vi "诊断标定4.vi"(8 "CAN端口":u16(ring), 9 "设备索引号":u16(ring), 10 "CAN卡类型":u32(ring)=4) -> ()   [LabVIEW 2013] (continued)
            n2546 = property on="电流步长" class="DigNum (严格)"("Disabled"=w3724) -> ()  [unwired: 2 in, 2 out]
            n2547 = property on="SOC" class="DigNum (严格)"("Disabled"=0) -> ()  [unwired: 2 in, 2 out]
            n2548 = property on="充电总安时" class="DigNum (严格)"("Disabled"=w3723) -> ()  [unwired: 2 in, 2 out]
            n2549 = property on="放电总这时" class="DigNum (严格)"("Disabled"=w3723) -> ()  [unwired: 2 in, 2 out]
            n2550 = Not(x=w3731) -> (.not. x?=w3730:bool)
          }
          frame "车牌号" {
            w3734 = 2
            w3735 = 2
            w3737 = 2
            w3739 = 2
            w3742 = FALSE ("1 6")
            n2551 = property on="电池类型" class="DigNum (严格)"("Disabled"=w3739) -> ()  [unwired: 2 in, 2 out]
            n2552 = property on="电池厂家" class="DigNum (严格)"("Disabled"=w3739) -> ()  [unwired: 2 in, 2 out]
            n2553 = property on="电池地区" class="DigNum (严格)"("Disabled"=w3739) -> ()  [unwired: 2 in, 2 out]
            n2554 = property on="电池组序号" class="DigNum (严格)"("Disabled"=w3739) -> ()  [unwired: 2 in, 2 out]
            n2555 = property on="电池包串联数" class="DigNum (严格)"("Disabled"=w3739) -> ()  [unwired: 2 in, 2 out]
            n2556 = property on="电池包并联数" class="DigNum (严格)"("Disabled"=w3739) -> ()  [unwired: 2 in, 2 out]
            n2557 = property on="电池包安时数" class="DigNum (严格)"("Disabled"=w3739) -> ()  [unwired: 2 in, 2 out]
            n2558 = property on="电池组信息" class="Clust (严格)"("Disabled"=0) -> ()  [unwired: 2 in, 2 out]
            n2559 = property on="车牌号" class="Str"("Disabled"=0) -> ()  [unwired: 2 in, 2 out]
            n2560 = property on="电池包序号" class="DigNum (严格)"("Disabled"=2) -> ()  [unwired: 2 in, 2 out]
            n2561 = property on="充电次数" class="DigNum (严格)"("Disabled"=w3737) -> ()  [unwired: 2 in, 2 out]
            n2562 = property on="充满电时间" class="DigNum (严格)"("Disabled"=w3737) -> ()  [unwired: 2 in, 2 out]
            n2563 = property on="放空时间" class="DigNum (严格)"("Disabled"=w3737) -> ()  [unwired: 2 in, 2 out]
            n2564 = property on="最大允许单体电压" class="DigNum (严格)"("Disabled"=w3735) -> ()  [unwired: 2 in, 2 out]
            n2565 = property on="最大允许总电压" class="DigNum (严格)"("Disabled"=w3735) -> ()  [unwired: 2 in, 2 out]
            n2566 = property on="最大允许温度" class="DigNum (严格)"("Disabled"=w3735) -> ()  [unwired: 2 in, 2 out]
            n2567 = property on="最小允许温度" class="DigNum (严格)"("Disabled"=w3735) -> ()  [unwired: 2 in, 2 out]
            n2568 = property on="最大允许充电电流" class="DigNum (严格)"("Disabled"=w3735) -> ()  [unwired: 2 in, 2 out]
            n2569 = property on="最小允许充电电流" class="DigNum (严格)"("Disabled"=w3735) -> ()  [unwired: 2 in, 2 out]
            n2570 = property on="最小允许单体电压" class="DigNum (严格)"("Disabled"=w3735) -> ()  [unwired: 2 in, 2 out]
            n2571 = property on="电流步长" class="DigNum (严格)"("Disabled"=w3735) -> ()  [unwired: 2 in, 2 out]
            n2572 = property on="SOC" class="DigNum (严格)"("Disabled"=2) -> ()  [unwired: 2 in, 2 out]
            n2573 = property on="充电总安时" class="DigNum (严格)"("Disabled"=w3734) -> ()  [unwired: 2 in, 2 out]
            n2574 = property on="放电总这时" class="DigNum (严格)"("Disabled"=w3734) -> ()  [unwired: 2 in, 2 out]
            n2575 = Not(x=w3742) -> (.not. x?=w3741:bool)
          }
          frame "充电参数" {
            w3744 = 2
            w3745 = 0
            w3747 = 2
            w3749 = 2
            w3752 = FALSE ("1 6")
            n2576 = property on="电池类型" class="DigNum (严格)"("Disabled"=w3749) -> ()  [unwired: 2 in, 2 out]
            n2577 = property on="电池厂家" class="DigNum (严格)"("Disabled"=w3749) -> ()  [unwired: 2 in, 2 out]
            n2578 = property on="电池地区" class="DigNum (严格)"("Disabled"=w3749) -> ()  [unwired: 2 in, 2 out]
            n2579 = property on="电池组序号" class="DigNum (严格)"("Disabled"=w3749) -> ()  [unwired: 2 in, 2 out]
            n2580 = property on="电池包串联数" class="DigNum (严格)"("Disabled"=w3749) -> ()  [unwired: 2 in, 2 out]
            n2581 = property on="电池包并联数" class="DigNum (严格)"("Disabled"=w3749) -> ()  [unwired: 2 in, 2 out]
            n2582 = property on="电池包安时数" class="DigNum (严格)"("Disabled"=w3749) -> ()  [unwired: 2 in, 2 out]
            n2583 = property on="电池组信息" class="Clust (严格)"("Disabled"=0) -> ()  [unwired: 2 in, 2 out]
            n2584 = property on="车牌号" class="Str"("Disabled"=2) -> ()  [unwired: 2 in, 2 out]
            n2585 = property on="电池包序号" class="DigNum (严格)"("Disabled"=2) -> ()  [unwired: 2 in, 2 out]
            n2586 = property on="充电次数" class="DigNum (严格)"("Disabled"=w3747) -> ()  [unwired: 2 in, 2 out]
            n2587 = property on="充满电时间" class="DigNum (严格)"("Disabled"=w3747) -> ()  [unwired: 2 in, 2 out]
            n2588 = property on="放空时间" class="DigNum (严格)"("Disabled"=w3747) -> ()  [unwired: 2 in, 2 out]
            n2589 = property on="最大允许单体电压" class="DigNum (严格)"("Disabled"=w3745) -> ()  [unwired: 2 in, 2 out]
            n2590 = property on="最大允许总电压" class="DigNum (严格)"("Disabled"=w3745) -> ()  [unwired: 2 in, 2 out]
            n2591 = property on="最大允许温度" class="DigNum (严格)"("Disabled"=w3745) -> ()  [unwired: 2 in, 2 out]
            n2592 = property on="最小允许温度" class="DigNum (严格)"("Disabled"=w3745) -> ()  [unwired: 2 in, 2 out]
            n2593 = property on="最大允许充电电流" class="DigNum (严格)"("Disabled"=w3745) -> ()  [unwired: 2 in, 2 out]
            n2594 = property on="最小允许充电电流" class="DigNum (严格)"("Disabled"=w3745) -> ()  [unwired: 2 in, 2 out]
            n2595 = property on="最小允许单体电压" class="DigNum (严格)"("Disabled"=w3745) -> ()  [unwired: 2 in, 2 out]
            n2596 = property on="电流步长" class="DigNum (严格)"("Disabled"=w3745) -> ()  [unwired: 2 in, 2 out]
            n2597 = property on="SOC" class="DigNum (严格)"("Disabled"=w3744) -> ()  [unwired: 2 in, 2 out]
            n2598 = property on="充电总安时" class="DigNum (严格)"("Disabled"=w3744) -> ()  [unwired: 2 in, 2 out]
            n2599 = property on="放电总这时" class="DigNum (严格)"("Disabled"=w3744) -> ()  [unwired: 2 in, 2 out]
            n2600 = Not(x=w3752) -> (.not. x?=w3751:bool)
          }
          frame "假", Default {
            w3755 = FALSE ("1 6")
            n2601 = Not(x=w3755) -> (.not. x?=w3754:bool)
          }
        }
        n2602 = local write "等级 2"(w3505) -> ()
        n2603 = local write "1 6"(w3504) -> ()
        n2604 = local write "1 7"(w3503) -> ()
        n2605 = local write "1 8"(w3502) -> ()
        n2606 = local write "1 9"(w3501) -> ()
        n2607 = local write "1 10"(w3500) -> ()
        n2608 = property on="单个读取" class="Bool (严格)"("Visible"=w3499) -> ()  [unwired: 2 in, 2 out]
        n2609 = property on="单个写入" class="Bool (严格)"("Visible"=w3498) -> ()  [unwired: 2 in, 2 out]
      }
      event "从板个数": Value Change {
        n2610 = event-data() -> ()  [unwired: 7 out]
        n2611 = local read "从板个数"() -> (w3757:dbl)
        n2612 = call "多从板对应参数.vi"("从板个数"=w3757) -> ("输出数组"=w3758:string[])  [unwired: 1 in]
        n2613 = control-ref of="项目信息"() -> (w3759:refnum<vi>)
        n2614 = stacked-sequence {
          tunnel: w3759 -> [w3762 w3766 w3770]
          tunnel: w3758 -> [_ w3765 w3769]
          frame #0 {
            n2615 = invoke class="Tbl (严格)" method="Reinit To Default"(reference=w3762) -> ()  [unwired: 2 in, 3 out]
          }
          frame #1 {
            n2616 = call "表格数据输入-8.6.vi"("行数"=u32 0, "列数"=u32 0, "字符串数组"=w3765, "表格引用"=w3766) -> ()  [unwired: 8 out]
          }
          frame #2 {
            n2617 = Array Size(array=w3769) -> (size(s)=w3768:i32)
            n2618 = for {
              N: w3768 -> [_]
              tunnel: [""] -> w3767 mode=indexing
            }
            n2619 = call "表格数据输入-8.6.vi"("行数"=u32 0, "列数"=u32 1, "字符串数组"=w3767, "表格引用"=w3770) -> ()  [unwired: 8 out]
          }
        }
      }
      event "主界面选项": Value Change {
        n2620 = event-data() -> ("NewVal"=w3774:enum32{"单选选项1", "单选选项2", "单选选项2 2", "单选选项2 3"})  [unwired: 6 out]
        n2621 = control-ref of="单选选项2 2"() -> (w3779:refnum<vi>)
        n2622 = control-ref of="单选选项2"() -> (w3781:refnum<vi>)
        n2623 = control-ref of="单选选项1"() -> (w3780:refnum<vi>)
        n2624 = control-ref of="单选选项2 3"() -> (w3775:refnum<vi>)
        n2625 = Build Array(w3780, w3781, w3779, w3775) -> (w3778:refnum<vi>[])
        n2626 = case shown="\"单选选项2 3\"" w3774 {
          selector: w3774 -> [w3792 w3797 w3802 w3807]
          tunnel: w3778 -> [w3793 w3798 w3803 w3808]
          tunnel: [w3791 w3796 w3801 w3806] -> w3784
          tunnel: [w3790 w3795 w3800 w3805] -> w3783
          tunnel: [enum32{"读写参数", "版本读取", "其它诊断"}."读写参数" ("选项卡控件 2") enum32{"读写参数", "版本读取", "其它诊断"}."版本读取" ("选项卡控件 2") enum32{"读写参数", "版本读取", "其它诊断"}."其它诊断" ("选项卡控件 2") enum32{"读写参数", "版本读取", "其它诊断", "高压板校正"}."高压板校正" ("选项卡控件 2")] -> w3782
          frame "单选选项1", Default {
            n2627 = Delete From Array(array=w3793, index=w3792) -> (deleted portion=w3790:refnum<vi>, array with subset deleted=w3791:refnum<vi>[])  [unwired: 1 in]
          }
          frame "单选选项2" {
            n2628 = Delete From Array(array=w3798, index=w3797) -> (deleted portion=w3795:refnum<vi>, array with subset deleted=w3796:refnum<vi>[])  [unwired: 1 in]
          }
          frame "单选选项2 2" {
            n2629 = Delete From Array(array=w3803, index=w3802) -> (deleted portion=w3800:refnum<vi>, array with subset deleted=w3801:refnum<vi>[])  [unwired: 1 in]
          }
          frame "单选选项2 3" {
            n2630 = Delete From Array(array=w3808, index=w3807) -> (deleted portion=w3805:refnum<vi>, array with subset deleted=w3806:refnum<vi>[])  [unwired: 1 in]
          }
        }
        n2631 = local write "选项卡控件 2"(w3782) -> ()
        n2632 = for {
          tunnel: u32 16777215 -> [w3788]
          tunnel: w3784 -> [w3787] mode=indexing
          n2633 = property class="Bool (严格)"(reference=w3787, "BoolText.TextColor"=w3788) -> ()  [unwired: 1 in, 2 out]
        }
        n2634 = property class="Bool (严格)"(reference=w3783, "BoolText.TextColor"=u32 87470) -> ()  [unwired: 1 in, 2 out]
      }
      event "主从板": Value Change {
        n2635 = event-data() -> ()  [unwired: 7 out]
        n2636 = control-ref of="单选选项2"() -> (w3816:refnum<vi>)
        n2637 = control-ref of="单选选项1"() -> (w3815:refnum<vi>)
        n2638 = local read "主从板"() -> (w3823:enum32{"单选选项2", "单选选项1"})
        n2639 = Build Array(w3816, w3815) -> (w3822:refnum<vi>[])
        n2640 = case shown="\"单选选项2\"" w3823 {
          selector: w3823 -> [w3867 w3892]
          tunnel: w3822 -> [w3868 w3891]
          tunnel: [enum32{"主板", "从板"}."主板" ("主从选择") enum32{"主板", "从板"}."从板" ("主从选择")] -> w3821
          tunnel: [w3866 w3890] -> w3818
          tunnel: [w3865 w3889] -> w3817
          tunnel: [TRUE FALSE] -> w3813
          tunnel: [w3826 w3869] -> w3810
          tunnel: [w3827 w3874] -> w3809
          frame "单选选项1", Default {
            n2641 = global read "功能码全局.vi" "主板项目信息7"() -> (w3838:bool[])
            n2642 = global read "功能码全局.vi" "主板控制类信息10"() -> (w3842:bool[])
            n2643 = global read "功能码全局.vi" "主板故障阀值9"() -> (w3839:bool[])
            n2644 = global read "功能码全局.vi" "主板项目信息5"() -> (w3852:bool[])
            n2645 = global read "功能码全局.vi" "主板项目信息6"() -> (w3862:bool[])
            n2646 = global read "功能码全局.vi" "主板项目信息4"() -> (w3861:bool[])
            n2647 = global read "功能码全局.vi" "主板版本号11"() -> (w3853:bool[])
            n2648 = Delete From Array(array=w3862, length=1 ("长度"), index=0 ("索引")) -> (deleted portion=w3851:bool[], array with subset deleted=w3834:bool[])
            n2649 = Index Array(array=w3861, index #1=5 ("索引"), index #2=6 ("索引")) -> (element #1=w3850:bool, element #2=w3833:bool)
            n2650 = Index Array(array=w3853) -> (element #1=w3846:bool, element #2=w3829:bool)  [unwired: 2 in]
            n2651 = Array Subset(array=w3839, index=2 ("索引"), length=3 ("长度")) -> (w3848:bool[])
            n2652 = Delete From Array(array=w3838, length=3 ("索引"), index=2 ("长度")) -> (deleted portion=w3849:bool[], array with subset deleted=w3832:bool[])
            n2653 = Array Subset(array=w3842, index=4 ("索引"), length=2 ("长度")) -> (w3847:bool[])
            n2654 = Delete From Array(array=w3868, index=w3867) -> (deleted portion=w3865:refnum<vi>, array with subset deleted=w3866:refnum<vi>[])  [unwired: 1 in]
            n2655 = Insert Into Array(array=w3852, new element #1=w3851, new element #2=w3850, new element #3=w3849, new element #4=w3848, new element #5=w3847, new element #6=w3846) -> (w3845:bool[])  [unwired: 1 in]
            n2656 = Array Subset(array=w3842, index=6 ("索引"), length=2 ("长度")) -> (w3830:bool[])
            n2657 = Array Subset(array=w3839, index=5 ("索引"), length=3 ("长度")) -> (w3831:bool[])
            n2658 = And Array Elements(Boolean array=w3845) -> (logical AND=w3827:bool)
            n2659 = Insert Into Array(array=w3834, new element #1=w3833, new element #2=w3832, new element #3=w3831, new element #4=w3830, new element #5=w3829) -> (w3828:bool[])  [unwired: 1 in]
            n2660 = And Array Elements(Boolean array=w3828) -> (logical AND=w3826:bool)
          }
          frame "单选选项2" {
            n2661 = global read "功能码全局.vi" "15"() -> (w3886:bool[])
            n2662 = global read "功能码全局.vi" "16"() -> (w3883:bool[])
            n2663 = Delete From Array(array=w3891, index=w3892) -> (deleted portion=w3889:refnum<vi>, array with subset deleted=w3890:refnum<vi>[])  [unwired: 1 in]
            n2664 = Index Array(array=w3883, index #1=4 ("索引"), index #2=5 ("索引"), index #3=6 ("索引"), index #4=7 ("索引")) -> (element #1=w3877:bool, element #2=w3876:bool, element #3=w3872:bool, element #4=w3871:bool)
            n2665 = Delete From Array(array=w3886, length=4 ("长度"), index=0 ("索引")) -> (deleted portion=w3878:bool[], array with subset deleted=w3873:bool[])
            n2666 = Insert Into Array(array=w3873, new element #1=w3872, new element #2=w3871) -> (w3870:bool[])  [unwired: 1 in]
            n2667 = Insert Into Array(array=w3878, new element #1=w3877, new element #2=w3876) -> (w3875:bool[])  [unwired: 1 in]
            n2668 = And Array Elements(Boolean array=w3870) -> (logical AND=w3869:bool)
            n2669 = And Array Elements(Boolean array=w3875) -> (logical AND=w3874:bool)
          }
        }
        n2670 = property on="全部写入" class="Bool (严格)"("Visible"=w3810) -> ()  [unwired: 2 in, 2 out]
        n2671 = property on="全部读取" class="Bool (严格)"("Visible"=w3809) -> ()  [unwired: 2 in, 2 out]
        n2672 = property on="从板个数" class="DigNum (严格)"("Visible"=w3813) -> ()  [unwired: 2 in, 2 out]
        n2673 = local write "主从选择"(w3821) -> ()
        n2674 = for {
          tunnel: u32 87470 -> [w3825]
          tunnel: w3818 -> [w3824] mode=indexing
          n2675 = property class="Bool (严格)"(reference=w3824, "BoolText.TextColor"=w3825) -> ()  [unwired: 1 in, 2 out]
        }
        n2676 = Not(x=w3813) -> (.not. x?=w3814:bool)
        n2677 = property class="Bool (严格)"(reference=w3817, "BoolText.TextColor"=u32 16777215) -> ()  [unwired: 1 in, 2 out]
        n2678 = property on="主板选项" class="Tree (严格)"("Visible"=w3813) -> ()  [unwired: 2 in, 2 out]
        n2679 = property on="从板选项" class="Tree (严格)"("Visible"=w3814) -> ()  [unwired: 2 in, 2 out]
        n2680 = property on="当前从板板号" class="DigNum (严格)"("Visible"=w3814) -> ()  [unwired: 2 in, 2 out]
      }
      event "从板板号": Value Change {
        n2681 = event-data() -> ()  [unwired: 7 out]
        n2682 = local read "key names"() -> (w3894:string[])
        n2683 = Empty Array?(array=w3894) -> (empty?=w3893:bool)
        n2684 = case shown="假" w3893 {
          tunnel: w3894 -> [w3897 _]
          frame False {
            n2685 = stacked-sequence {
              seq-local: [w3898 _] -> [_ w3961]
              tunnel: w3897 -> [w3906 _]
              frame #0 {
                w3937 = 2 ("长度")
                w3934 = 20 ("长度")
                w3922 = 1 ("索引")
                n2686 = local read "从板板号"() -> (w3898:u8)
                n2687 = local read "输出数组"() -> (w3907:string[][])
                n2688 = Decrement(x=w3898) -> (x-1=w3904:u8)
                n2689 = Index Array(array=w3907, index (col)=w3904) -> (element=w3935:string[])  [unwired: 1 in]
                n2690 = global write "读配置文件全局2.vi" "从板板号"(w3898) -> ()
                n2691 = Search 1D Array(1D array=w3906, element="风机开启温度" ("元素")) -> (index of element=w3919:i32)  [unwired: 1 in]
                n2692 = Search 1D Array(1D array=w3906, element="电压过高一级" ("元素"), start index (0)=w3919) -> (index of element=w3917:i32)
                n2693 = Decrement(x=w3919) -> (x-1=w3921:i32)
                n2694 = Array Subset(array=w3935, index=w3922, length=w3921) -> (w3905:string[])
                n2695 = Array Subset(array=w3935, index=w3917, length=21 ("长度")) -> (w3909:string[])
                n2696 = Array Subset(array=w3906, index=w3922, length=w3921) -> (w3952:string[])
                n2697 = Array Subset(array=w3935, index=w3919, length=7 ("长度")) -> (w3915:string[])
                n2698 = for {
                  tunnel: w3909 -> [w3954] mode=indexing
                  tunnel: [w3953] -> w3908 mode=indexing
                  n2699 = Fract/Exp String To Number(string=w3954) -> (number=w3953:dbl)  [unwired: 3 in, 1 out]
                }
                n2700 = for {
                  tunnel: w3915 -> [w3956] mode=indexing
                  tunnel: [w3955] -> w3899 mode=indexing
                  n2701 = Fract/Exp String To Number(string=w3956) -> (number=w3955:dbl)  [unwired: 3 in, 1 out]
                }
                n2702 = Delete From Array(array=w3908, length=7 ("长度"), index=0 ("索引")) -> (deleted portion=w3902:dbl[], array with subset deleted=w3912:dbl[])
                n2703 = Array To Cluster(array=w3899) -> (cluster=w3924:T23)
                n2704 = global write "读配置文件全局2.vi" "加热控制参数"(w3899) -> ()
                n2705 = Delete From Array(array=w3912, length=7 ("长度"), index=0 ("索引")) -> (deleted portion=w3901:dbl[], array with subset deleted=w3900:dbl[])
                n2706 = local write "加热控制参数"(w3924) -> ()
                n2707 = Array To Cluster(array=w3902) -> (cluster=w3949:T23)
                n2708 = Array To Cluster(array=w3900) -> (cluster=w3951:T23)
                n2709 = Array To Cluster(array=w3901) -> (cluster=w3950:T23)
                n2710 = global write "读配置文件全局2.vi" "三级故障阀值"(w3900) -> ()
                n2711 = global write "读配置文件全局2.vi" "一级故障阀值"(w3902) -> ()
                n2712 = global write "读配置文件全局2.vi" "二级故障阀值"(w3901) -> ()
                n2713 = local write "一级故障 6"(w3949) -> ()
                n2714 = local write "一级故障 8"(w3951) -> ()
                n2715 = local write "一级故障 7"(w3950) -> ()
                n2716 = Search 1D Array(1D array=w3952, element="温度个数" ("元素")) -> (index of element=w3931:i32)  [unwired: 1 in]
                n2717 = Search 1D Array(1D array=w3952, element="第一个保险通道" ("元素")) -> (index of element=w3932:i32)  [unwired: 1 in]
                n2718 = Search 1D Array(1D array=w3952, element="电压个数" ("元素")) -> (index of element=w3930:i32)  [unwired: 1 in]
                n2719 = Search 1D Array(1D array=w3952, element="第1通道电压个数" ("元素")) -> (index of element=w3933:i32)  [unwired: 1 in]
                n2720 = Array Subset(array=w3905, index=w3930, length=2 ("长度")) -> (w3938:string[])
                n2721 = Array Subset(array=w3905, index=w3931, length=w3937) -> (w3940:string[])
                n2722 = Array Subset(array=w3905, index=w3932, length=20 ("长度")) -> (w3941:string[])
                n2723 = Array Subset(array=w3905, index=w3933, length=w3934) -> (w3939:string[])
                n2724 = Insert Into Array(array=w3938, new element #1=w3939, new element #2=w3940, new element #3=w3941) -> (w3903:string[])  [unwired: 1 in]
                n2725 = Array Subset(array=w3952, index=w3930, length=w3937) -> (w3942:string[])
                n2726 = Array Subset(array=w3952, index=w3931, length=w3937) -> (w3944:string[])
                n2727 = Array Subset(array=w3952, index=w3932, length=w3934) -> (w3945:string[])
                n2728 = Array Subset(array=w3952, index=w3933, length=w3934) -> (w3943:string[])
                n2729 = global write "读配置文件全局2.vi" "表格"(w3903) -> ()
                n2730 = Insert Into Array(array=w3942, new element #1=w3943, new element #2=w3944, new element #3=w3945) -> (w3947:string[])  [unwired: 1 in]
                n2731 = Build Array(w3947, w3903) -> (w3946:string[][])
                n2732 = Transpose 2D Array(2D array=w3946) -> (transposed array=w3948:string[][])
                n2733 = local write "项目信息 2"(w3948) -> ()
              }
              frame #1 {
                n2734 = Number To Decimal String(number=w3961) -> (decimal integer string=w3959:string)  [unwired: 1 in]
                n2735 = control-ref of="结果"() -> (w3964:refnum<vi>)
                n2736 = Concatenate Strings("从板", w3959, "导入完成") -> (w3957:string)
                n2737 = Build Array(w3957) -> (w3962:string[])
                n2738 = call "表格编辑.vi"("新元素/子数组"=w3962, "活动单元格:单元格背景色"=u32 6618880, "MCListbox引用句柄"=w3964) -> ()  [unwired: 9 out]
              }
            }
          }
          frame True {
          }
        }
      }
      event "读配置文件": Value Change {
        n2739 = event-data() -> ("NewVal"=w3965:bool)  [unwired: 6 out]
        n2740 = case shown="真" w3965 {
          tunnel: w3969 -> [w3971 w3977]
          tunnel: [w3971 w3976] -> w3968
          tunnel: w3967 -> [w3970 w3975]
          tunnel: [w3970 w3974] -> w3966
          frame False {
          }
          frame True {
            n2741 = local write "布尔"(TRUE ("布尔")) -> ()
            n2742 = Enqueue Element(queue=w3977, element="读配置文件", error in (no error)=w3975) -> (queue out=w3976:refnum<queue>, error out=w3974:errorcluster)  [unwired: 2 out]
            n2743 = call <vilib>:"Set Busy.vi"() -> ()  [unwired: 4 in, 8 out]
          }
        }
      }
      event "写配置文件": Value Change {
        n2744 = event-data() -> ("NewVal"=w3978:bool)  [unwired: 6 out]
        n2745 = case shown="真" w3978 {
          tunnel: w3982 -> [w3984 w3989]
          tunnel: [w3984 w3988] -> w3981
          tunnel: w3980 -> [w3983 w3987]
          tunnel: [w3983 w3986] -> w3979
          frame False {
          }
          frame True {
            n2746 = call <vilib>:"Set Busy.vi"() -> ()  [unwired: 4 in, 8 out]
            n2747 = Enqueue Element(queue=w3989, element="写配置文件", error in (no error)=w3987) -> (queue out=w3988:refnum<queue>, error out=w3986:errorcluster)  [unwired: 2 out]
          }
        }
      }
      event "继电器全开": Value Change {
        n2748 = event-data() -> ("NewVal"=w3990:bool)  [unwired: 6 out]
        n2749 = stacked-sequence {
          tunnel: w3990 -> [_ w4000 _]
          frame #0 {
            w3993 = FALSE ("清BUFF")
            n2750 = local write "继电器超时处理"(FALSE ("继电器超时处理")) -> ()
            n2751 = local write "主从选择"(enum32{"主板", "从板"}."主板" ("主从选择")) -> ()
            n2752 = local write "正级继电器 12"(w3993) -> ()
            n2753 = local write "清BUFF"(w3993) -> ()
            n2754 = local write "正级继电器 2"(w3993) -> ()
            n2755 = local write "正级继电器 3"(w3993) -> ()
            n2756 = local write "正级继电器 4"(w3993) -> ()
            n2757 = local write "正级继电器 5"(w3993) -> ()
            n2758 = local write "正级继电器 6"(w3993) -> ()
          }
          frame #1 {
            n2759 = case shown="真" w4000 {
              selector: w4000 -> [_ w4015]
              frame False {
              }
              frame True {
                w4011 = 256.0 ("y")
                w4002 = u32 1 ("命令序号")
                w4001 = u8 192 ("命令")
                n2760 = local read "动作保持时间"() -> (w4012:dbl)
                n2761 = Quotient & Remainder(x=w4012, y=w4011) -> (x-y*floor(x/y)=w4004:dbl, floor(x/y)=w4008:dbl)
                n2762 = Quotient & Remainder(x=w4008, y=w4011) -> (x-y*floor(x/y)=w4005:dbl, floor(x/y)=w4009:dbl)
                n2763 = local read "设备索引号"() -> (w4019:u16)
                n2764 = Quotient & Remainder(x=w4009, y=w4011) -> (x-y*floor(x/y)=w4006:dbl, floor(x/y)=w4010:dbl)
                n2765 = local read "CAN卡类型"() -> (w4020:u32)
                n2766 = local read "CAN端口"() -> (w4018:u16)
                n2767 = Boolean To (0,1)(Boolean=w4015) -> (0, 1=w4013:i16)
                n2768 = Quotient & Remainder(x=w4010, y=w4011) -> (x-y*floor(x/y)=w4007:dbl)  [unwired: 1 out]
                n2769 = Build Array(i16 170 ("元素"), w4013, w4007, w4006, w4005, w4004, 0.0 ("元素")) -> (w4016:dbl[])
                n2770 = call "多帧发送机制(EV05).vi"("can卡类型"=w4020, "设备索引号"=w4019, "CAN端口"=w4018, "命令"=w4001, "板号"=u8 0, "命令序号"=w4002, "输入数据"=w4016) -> ()  [unwired: 1 in, 12 out]
                n2771 = local write "命令序号"(w4002) -> ()
                n2772 = local write "命令"(w4001) -> ()
              }
            }
            n2773 = local write "控制1"(TRUE ("控制1")) -> ()
            n2774 = local write "写?"(FALSE ("写?")) -> ()
            n2775 = global write "EV05全局变量1.vi" "流控帧 2"(FALSE ("流控帧 2")) -> ()
            n2776 = local write "消除"(TRUE ("消除")) -> ()
          }
          frame #2 {
            n2777 = flat-sequence {
              tunnel: [w4022] -> w4021
              tunnel: w4021 -> [w4029]
              frame #0 {
                n2778 = while {
                  tunnel: [w4023] -> w4022
                  i -> [w4027]
                  stop <- w4024 stop-if-true
                  n2779 = local read "继电器超时处理"() -> (w4023:bool)
                  n2780 = Greater Or Equal?(x=w4027, y=20) -> (x >= y?=w4025:bool)
                  n2781 = Wait Until Next ms Multiple(millisecond multiple=u32 100 ("毫秒倍数")) -> ()  [unwired: 1 out]
                  n2782 = Or(x=w4023, y=w4025) -> (x .or. y?=w4024:bool)
                }
              }
              frame #1 {
                n2783 = case shown="假" w4029 {
                  frame False {
                    n2784 = One Button Dialog(message="继电器处理超时" ("消息"), button name ("OK")="是" ("按钮名称（“确定”）")) -> ()  [unwired: 1 out]
                  }
                  frame True {
                    w4032 = TRUE ("清BUFF")
                    n2785 = local write "正级继电器 12"(w4032) -> ()
                    n2786 = local write "正级继电器 2"(w4032) -> ()
                    n2787 = local write "正级继电器 3"(w4032) -> ()
                    n2788 = local write "正级继电器 4"(w4032) -> ()
                    n2789 = local write "正级继电器 5"(w4032) -> ()
                    n2790 = local write "正级继电器 6"(w4032) -> ()
                  }
                }
              }
            }
          }
        }
      }
      event "继电器全关": Value Change {
        n2791 = event-data() -> ("NewVal"=w4033:bool)  [unwired: 6 out]
        n2792 = stacked-sequence {
          tunnel: w4033 -> [_ w4044 _]
          frame #0 {
            w4036 = TRUE ("清BUFF")
            n2793 = local write "正级继电器 12"(w4036) -> ()
            n2794 = local write "正级继电器 2"(w4036) -> ()
            n2795 = local write "正级继电器 3"(w4036) -> ()
            n2796 = local write "正级继电器 4"(w4036) -> ()
            n2797 = local write "正级继电器 5"(w4036) -> ()
            n2798 = local write "正级继电器 6"(w4036) -> ()
            n2799 = local write "继电器超时处理"(FALSE ("继电器超时处理")) -> ()
            n2800 = local write "主从选择"(enum32{"主板", "从板"}."主板" ("主从选择")) -> ()
            n2801 = local write "清BUFF"(FALSE ("清BUFF")) -> ()
          }
          frame #1 {
            n2802 = case shown="真" w4044 {
              selector: w4044 -> [_ w4059]
              frame False {
              }
              frame True {
                w4055 = 256.0 ("y")
                w4046 = u32 1 ("命令序号")
                w4045 = u8 192 ("命令")
                n2803 = local read "动作保持时间"() -> (w4056:dbl)
                n2804 = Quotient & Remainder(x=w4056, y=w4055) -> (x-y*floor(x/y)=w4048:dbl, floor(x/y)=w4052:dbl)
                n2805 = Quotient & Remainder(x=w4052, y=w4055) -> (x-y*floor(x/y)=w4049:dbl, floor(x/y)=w4053:dbl)
                n2806 = local read "设备索引号"() -> (w4063:u16)
                n2807 = Quotient & Remainder(x=w4053, y=w4055) -> (x-y*floor(x/y)=w4050:dbl, floor(x/y)=w4054:dbl)
                n2808 = local read "CAN卡类型"() -> (w4064:u32)
                n2809 = local read "CAN端口"() -> (w4062:u16)
                n2810 = Boolean To (0,1)(Boolean=w4059) -> (0, 1=w4057:i16)
                n2811 = Quotient & Remainder(x=w4054, y=w4055) -> (x-y*floor(x/y)=w4051:dbl)  [unwired: 1 out]
                n2812 = Build Array(i16 85 ("元素"), w4057, w4051, w4050, w4049, w4048, 0.0 ("元素")) -> (w4060:dbl[])
                n2813 = call "多帧发送机制(EV05).vi"("can卡类型"=w4064, "设备索引号"=w4063, "CAN端口"=w4062, "命令"=w4045, "板号"=u8 0, "命令序号"=w4046, "输入数据"=w4060) -> ()  [unwired: 1 in, 12 out]
                n2814 = local write "命令序号"(w4046) -> ()
                n2815 = local write "命令"(w4045) -> ()
              }
            }
            n2816 = local write "控制1"(TRUE ("控制1")) -> ()
            n2817 = local write "写?"(FALSE ("写?")) -> ()
            n2818 = global write "EV05全局变量1.vi" "流控帧 2"(FALSE ("流控帧 2")) -> ()
            n2819 = local write "消除"(TRUE ("消除")) -> ()
          }
          frame #2 {
            n2820 = flat-sequence {
              tunnel: [w4066] -> w4065
              tunnel: w4065 -> [w4073]
              frame #0 {
                n2821 = while {
                  tunnel: [w4067] -> w4066
                  i -> [w4071]
                  stop <- w4068 stop-if-true
                  n2822 = local read "继电器超时处理"() -> (w4067:bool)
                  n2823 = Greater Or Equal?(x=w4071, y=20) -> (x >= y?=w4069:bool)
                  n2824 = Wait Until Next ms Multiple(millisecond multiple=u32 100 ("毫秒倍数")) -> ()  [unwired: 1 out]
                  n2825 = Or(x=w4067, y=w4069) -> (x .or. y?=w4068:bool)
                }
              }
              frame #1 {
                n2826 = case shown="真" w4073 {
                  frame False {
                    n2827 = One Button Dialog(message="继电器处理超时" ("消息"), button name ("OK")="是" ("按钮名称（“确定”）")) -> ()  [unwired: 1 out]
                  }
                  frame True {
                    w4076 = FALSE ("清BUFF")
                    n2828 = local write "正级继电器 12"(w4076) -> ()
                    n2829 = local write "正级继电器 2"(w4076) -> ()
                    n2830 = local write "正级继电器 3"(w4076) -> ()
                    n2831 = local write "正级继电器 4"(w4076) -> ()
                    n2832 = local write "正级继电器 5"(w4076) -> ()
                    n2833 = local write "正级继电器 6"(w4076) -> ()
                  }
                }
              }
            }
          }
        }
      }
      event "控制按键全为开": Value Change {
        n2834 = event-data() -> ("NewVal"=w4077:bool)  [unwired: 6 out]
        n2835 = case shown="真" w4077 {
          frame False {
          }
          frame True {
            w4078 = TRUE ("正级继电器")
            n2836 = local write "DO1 2"(w4078) -> ()
            n2837 = local write "正级继电器"(w4078) -> ()
            n2838 = local write "负级继电器"(w4078) -> ()
            n2839 = local write "预充电继电器"(w4078) -> ()
            n2840 = local write "加热继电器"(w4078) -> ()
            n2841 = local write "加热继电器"(w4078) -> ()
            n2842 = local write "风机继电器"(w4078) -> ()
            n2843 = local write "DO1"(w4078) -> ()
            n2844 = local write "DO2"(w4078) -> ()
            n2845 = local write "充电继电器"(w4078) -> ()
            n2846 = local write "风机继电器"(w4078) -> ()
          }
        }
      }
      event "控制按键全为关": Value Change {
        n2847 = event-data() -> ("NewVal"=w4079:bool)  [unwired: 6 out]
        n2848 = case shown="真" w4079 {
          frame False {
          }
          frame True {
            w4080 = FALSE ("正级继电器")
            n2849 = local write "DO1 2"(w4080) -> ()
            n2850 = local write "正级继电器"(w4080) -> ()
            n2851 = local write "负级继电器"(w4080) -> ()
            n2852 = local write "预充电继电器"(w4080) -> ()
            n2853 = local write "加热继电器"(w4080) -> ()
            n2854 = local write "加热继电器"(w4080) -> ()
            n2855 = local write "风机继电器"(w4080) -> ()
            n2856 = local write "DO1"(w4080) -> ()
            n2857 = local write "DO2"(w4080) -> ()
            n2858 = local write "充电继电器"(w4080) -> ()
            n2859 = local write "风机继电器"(w4080) -> ()
          }
        }
      }
      event "正级继电器": Value Change {
        n2860 = event-data() -> ("NewVal"=w4081:bool)  [unwired: 6 out]
        n2861 = stacked-sequence {
          tunnel: w4081 -> [_ w4093 _]
          frame #0 {
            w4084 = FALSE ("清BUFF")
            n2862 = local write "继电器超时处理"(FALSE ("继电器超时处理")) -> ()
            n2863 = local write "主从选择"(enum32{"主板", "从板"}."主板" ("主从选择")) -> ()
            n2864 = local write "正级继电器 12"(w4084) -> ()
            n2865 = local write "清BUFF"(w4084) -> ()
          }
          frame #1 {
            n2866 = case shown="假" w4093 {
              selector: w4093 -> [w4108 w4128]
              tunnel: [w4107 w4127] -> w4092
              tunnel: [w4095 w4115] -> w4087
              frame False {
                w4103 = 256.0 ("y")
                w4095 = u32 1 ("命令序号")
                w4107 = u8 192 ("命令")
                n2867 = local read "动作保持时间"() -> (w4104:dbl)
                n2868 = Quotient & Remainder(x=w4104, y=w4103) -> (x-y*floor(x/y)=w4096:dbl, floor(x/y)=w4100:dbl)
                n2869 = Quotient & Remainder(x=w4100, y=w4103) -> (x-y*floor(x/y)=w4097:dbl, floor(x/y)=w4101:dbl)
                n2870 = local read "设备索引号"() -> (w4112:u16)
                n2871 = Quotient & Remainder(x=w4101, y=w4103) -> (x-y*floor(x/y)=w4098:dbl, floor(x/y)=w4102:dbl)
                n2872 = local read "CAN卡类型"() -> (w4113:u32)
                n2873 = local read "CAN端口"() -> (w4111:u16)
                n2874 = Boolean To (0,1)(Boolean=w4108) -> (0, 1=w4105:i16)
                n2875 = Quotient & Remainder(x=w4102, y=w4103) -> (x-y*floor(x/y)=w4099:dbl)  [unwired: 1 out]
                n2876 = Build Array(i16 1 ("元素"), w4105, w4099, w4098, w4097, w4096, 0.0 ("元素")) -> (w4109:dbl[])
                n2877 = call "多帧发送机制(EV05).vi"("can卡类型"=w4113, "设备索引号"=w4112, "CAN端口"=w4111, "命令"=w4107, "板号"=u8 0, "命令序号"=w4095, "输入数据"=w4109) -> ()  [unwired: 1 in, 12 out]
              }
              frame True {
                w4123 = 256.0 ("y")
                w4115 = u32 1 ("命令序号")
                w4127 = u8 192 ("命令")
                n2878 = local read "动作保持时间"() -> (w4124:dbl)
                n2879 = Quotient & Remainder(x=w4124, y=w4123) -> (x-y*floor(x/y)=w4116:dbl, floor(x/y)=w4120:dbl)
                n2880 = Quotient & Remainder(x=w4120, y=w4123) -> (x-y*floor(x/y)=w4117:dbl, floor(x/y)=w4121:dbl)
                n2881 = local read "设备索引号"() -> (w4132:u16)
                n2882 = Quotient & Remainder(x=w4121, y=w4123) -> (x-y*floor(x/y)=w4118:dbl, floor(x/y)=w4122:dbl)
                n2883 = local read "CAN卡类型"() -> (w4133:u32)
                n2884 = local read "CAN端口"() -> (w4131:u16)
                n2885 = Boolean To (0,1)(Boolean=w4128) -> (0, 1=w4125:i16)
                n2886 = Quotient & Remainder(x=w4122, y=w4123) -> (x-y*floor(x/y)=w4119:dbl)  [unwired: 1 out]
                n2887 = Build Array(i16 1 ("元素"), w4125, w4119, w4118, w4117, w4116, 0.0 ("元素")) -> (w4129:dbl[])
                n2888 = call "多帧发送机制(EV05).vi"("can卡类型"=w4133, "设备索引号"=w4132, "CAN端口"=w4131, "命令"=w4127, "板号"=u8 0, "命令序号"=w4115, "输入数据"=w4129) -> ()  [unwired: 1 in, 12 out]
              }
            }
            n2889 = local write "命令序号"(w4087) -> ()
            n2890 = local write "命令"(w4092) -> ()
            n2891 = local write "控制1"(TRUE ("控制1")) -> ()
            n2892 = local write "写?"(FALSE ("写?")) -> ()
            n2893 = global write "EV05全局变量1.vi" "流控帧 2"(FALSE ("流控帧 2")) -> ()
            n2894 = local write "消除"(TRUE ("消除")) -> ()
          }
          frame #2 {
            n2895 = flat-sequence {
              tunnel: [w4135] -> w4134
              tunnel: w4134 -> [w4142]
              frame #0 {
                n2896 = while {
                  tunnel: [w4136] -> w4135
                  i -> [w4140]
                  stop <- w4137 stop-if-true
                  n2897 = local read "继电器超时处理"() -> (w4136:bool)
                  n2898 = Greater Or Equal?(x=w4140, y=20) -> (x >= y?=w4138:bool)
                  n2899 = Wait Until Next ms Multiple(millisecond multiple=u32 100 ("毫秒倍数")) -> ()  [unwired: 1 out]
                  n2900 = Or(x=w4136, y=w4138) -> (x .or. y?=w4137:bool)
                }
              }
              frame #1 {
                n2901 = case shown="假" w4142 {
                  frame False {
                    n2902 = local read "正级继电器"() -> (w4144:bool)
                    n2903 = Not(x=w4144) -> (.not. x?=w4143:bool)
                    n2904 = local write "正级继电器"(w4143) -> ()
                    n2905 = One Button Dialog(message="继电器处理超时" ("消息"), button name ("OK")="是" ("按钮名称（“确定”）")) -> ()  [unwired: 1 out]
                  }
                  frame True {
                  }
                }
              }
            }
          }
        }
      }
      event "负级继电器": Value Change {
        n2906 = event-data() -> ("NewVal"=w4147:bool)  [unwired: 6 out]
        n2907 = stacked-sequence {
          tunnel: w4147 -> [_ w4159 _]
          frame #0 {
            w4150 = FALSE ("继电器超时处理")
            n2908 = local write "继电器超时处理"(w4150) -> ()
            n2909 = local write "正级继电器 2"(w4150) -> ()
            n2910 = local write "主从选择"(enum32{"主板", "从板"}."主板" ("主从选择")) -> ()
          }
          frame #1 {
            n2911 = case shown="假" w4159 {
              selector: w4159 -> [w4173 w4193]
              tunnel: [w4172 w4192] -> w4158
              tunnel: [w4161 w4181] -> w4153
              frame False {
                w4169 = 256.0 ("y")
                w4161 = u32 1 ("命令序号")
                w4172 = u8 192 ("命令")
                n2912 = local read "动作保持时间"() -> (w4170:dbl)
                n2913 = Quotient & Remainder(x=w4170, y=w4169) -> (x-y*floor(x/y)=w4162:dbl, floor(x/y)=w4166:dbl)
                n2914 = Quotient & Remainder(x=w4166, y=w4169) -> (x-y*floor(x/y)=w4163:dbl, floor(x/y)=w4167:dbl)
                n2915 = Quotient & Remainder(x=w4167, y=w4169) -> (x-y*floor(x/y)=w4164:dbl, floor(x/y)=w4168:dbl)
                n2916 = Quotient & Remainder(x=w4168, y=w4169) -> (x-y*floor(x/y)=w4165:dbl)  [unwired: 1 out]
                n2917 = Boolean To (0,1)(Boolean=w4173) -> (0, 1=w4171:i16)
                n2918 = local read "设备索引号"() -> (w4178:u16)
                n2919 = local read "CAN卡类型"() -> (w4179:u32)
                n2920 = local read "CAN端口"() -> (w4177:u16)
                n2921 = Build Array(i16 2 ("元素"), w4171, w4165, w4164, w4163, w4162, 0.0 ("元素")) -> (w4175:dbl[])
                n2922 = call "多帧发送机制(EV05).vi"("can卡类型"=w4179, "设备索引号"=w4178, "CAN端口"=w4177, "命令"=w4172, "板号"=u8 0, "命令序号"=w4161, "输入数据"=w4175) -> ()  [unwired: 1 in, 12 out]
              }
              frame True {
                w4189 = 256.0 ("y")
                w4181 = u32 1 ("命令序号")
                w4192 = u8 192 ("命令")
                n2923 = local read "动作保持时间"() -> (w4190:dbl)
                n2924 = Quotient & Remainder(x=w4190, y=w4189) -> (x-y*floor(x/y)=w4182:dbl, floor(x/y)=w4186:dbl)
                n2925 = Quotient & Remainder(x=w4186, y=w4189) -> (x-y*floor(x/y)=w4183:dbl, floor(x/y)=w4187:dbl)
                n2926 = Quotient & Remainder(x=w4187, y=w4189) -> (x-y*floor(x/y)=w4184:dbl, floor(x/y)=w4188:dbl)
                n2927 = Quotient & Remainder(x=w4188, y=w4189) -> (x-y*floor(x/y)=w4185:dbl)  [unwired: 1 out]
                n2928 = Boolean To (0,1)(Boolean=w4193) -> (0, 1=w4191:i16)
                n2929 = local read "设备索引号"() -> (w4198:u16)
                n2930 = local read "CAN卡类型"() -> (w4199:u32)
                n2931 = local read "CAN端口"() -> (w4197:u16)
                n2932 = Build Array(i16 2 ("元素"), w4191, w4185, w4184, w4183, w4182, 0.0 ("元素")) -> (w4195:dbl[])
                n2933 = call "多帧发送机制(EV05).vi"("can卡类型"=w4199, "设备索引号"=w4198, "CAN端口"=w4197, "命令"=w4192, "板号"=u8 0, "命令序号"=w4181, "输入数据"=w4195) -> ()  [unwired: 1 in, 12 out]
              }
            }
            n2934 = local write "命令"(w4158) -> ()
            n2935 = local write "命令序号"(w4153) -> ()
            n2936 = local write "清BUFF"(FALSE ("清BUFF")) -> ()
            n2937 = local write "控制1"(TRUE ("控制1")) -> ()
            n2938 = global write "EV05全局变量1.vi" "流控帧 2"(FALSE ("流控帧 2")) -> ()
            n2939 = local write "写?"(FALSE ("写?")) -> ()
            n2940 = local write "消除"(TRUE ("消除")) -> ()
          }
          frame #2 {
            n2941 = flat-sequence {
              tunnel: [w4201] -> w4200
              tunnel: w4200 -> [w4208]
              frame #0 {
                n2942 = while {
                  tunnel: [w4202] -> w4201
                  i -> [w4206]
                  stop <- w4203 stop-if-true
                  n2943 = local read "继电器超时处理"() -> (w4202:bool)
                  n2944 = Greater Or Equal?(x=w4206, y=20) -> (x >= y?=w4204:bool)
                  n2945 = Wait Until Next ms Multiple(millisecond multiple=u32 100 ("毫秒倍数")) -> ()  [unwired: 1 out]
                  n2946 = Or(x=w4202, y=w4204) -> (x .or. y?=w4203:bool)
                }
              }
              frame #1 {
                n2947 = case shown="假" w4208 {
                  frame False {
                    n2948 = local read "负级继电器"() -> (w4209:bool)
                    n2949 = Not(x=w4209) -> (.not. x?=w4210:bool)
                    n2950 = local write "负级继电器"(w4210) -> ()
                    n2951 = One Button Dialog(message="继电器处理超时" ("消息"), button name ("OK")="是" ("按钮名称（“确定”）")) -> ()  [unwired: 1 out]
                  }
                  frame True {
                  }
                }
              }
            }
          }
        }
      }
      event "预充电继电器": Value Change {
        n2952 = event-data() -> ("NewVal"=w4213:bool)  [unwired: 6 out]
        n2953 = stacked-sequence {
          tunnel: w4213 -> [_ w4225 _]
          frame #0 {
            w4216 = FALSE ("继电器超时处理")
            n2954 = local write "继电器超时处理"(w4216) -> ()
            n2955 = local write "正级继电器 3"(w4216) -> ()
            n2956 = local write "主从选择"(enum32{"主板", "从板"}."主板" ("主从选择")) -> ()
          }
          frame #1 {
            n2957 = case shown="假" w4225 {
              selector: w4225 -> [w4239 w4259]
              tunnel: [w4238 w4258] -> w4224
              tunnel: [w4227 w4247] -> w4219
              frame False {
                w4235 = 256.0 ("y")
                w4227 = u32 1 ("命令序号")
                w4238 = u8 192 ("命令")
                n2958 = local read "动作保持时间"() -> (w4236:dbl)
                n2959 = Quotient & Remainder(x=w4236, y=w4235) -> (x-y*floor(x/y)=w4228:dbl, floor(x/y)=w4232:dbl)
                n2960 = Quotient & Remainder(x=w4232, y=w4235) -> (x-y*floor(x/y)=w4229:dbl, floor(x/y)=w4233:dbl)
                n2961 = Quotient & Remainder(x=w4233, y=w4235) -> (x-y*floor(x/y)=w4230:dbl, floor(x/y)=w4234:dbl)
                n2962 = Quotient & Remainder(x=w4234, y=w4235) -> (x-y*floor(x/y)=w4231:dbl)  [unwired: 1 out]
                n2963 = Boolean To (0,1)(Boolean=w4239) -> (0, 1=w4237:i16)
                n2964 = local read "设备索引号"() -> (w4244:u16)
                n2965 = local read "CAN卡类型"() -> (w4245:u32)
                n2966 = local read "CAN端口"() -> (w4243:u16)
                n2967 = Build Array(i16 3 ("元素"), w4237, w4231, w4230, w4229, w4228, 0.0 ("元素")) -> (w4241:dbl[])
                n2968 = call "多帧发送机制(EV05).vi"("can卡类型"=w4245, "设备索引号"=w4244, "CAN端口"=w4243, "命令"=w4238, "板号"=u8 0, "命令序号"=w4227, "输入数据"=w4241) -> ()  [unwired: 1 in, 12 out]
              }
              frame True {
                w4255 = 256.0 ("y")
                w4247 = u32 1 ("命令序号")
                w4258 = u8 192 ("命令")
                n2969 = local read "动作保持时间"() -> (w4256:dbl)
                n2970 = Quotient & Remainder(x=w4256, y=w4255) -> (x-y*floor(x/y)=w4248:dbl, floor(x/y)=w4252:dbl)
                n2971 = Quotient & Remainder(x=w4252, y=w4255) -> (x-y*floor(x/y)=w4249:dbl, floor(x/y)=w4253:dbl)
                n2972 = Quotient & Remainder(x=w4253, y=w4255) -> (x-y*floor(x/y)=w4250:dbl, floor(x/y)=w4254:dbl)
                n2973 = Quotient & Remainder(x=w4254, y=w4255) -> (x-y*floor(x/y)=w4251:dbl)  [unwired: 1 out]
                n2974 = Boolean To (0,1)(Boolean=w4259) -> (0, 1=w4257:i16)
                n2975 = local read "设备索引号"() -> (w4264:u16)
                n2976 = local read "CAN卡类型"() -> (w4265:u32)
                n2977 = local read "CAN端口"() -> (w4263:u16)
                n2978 = Build Array(i16 3 ("元素"), w4257, w4251, w4250, w4249, w4248, 0.0 ("元素")) -> (w4261:dbl[])
                n2979 = call "多帧发送机制(EV05).vi"("can卡类型"=w4265, "设备索引号"=w4264, "CAN端口"=w4263, "命令"=w4258, "板号"=u8 0, "命令序号"=w4247, "输入数据"=w4261) -> ()  [unwired: 1 in, 12 out]
              }
            }
            n2980 = local write "命令序号"(w4219) -> ()
            n2981 = local write "清BUFF"(FALSE ("清BUFF")) -> ()
            n2982 = local write "控制1"(TRUE ("控制1")) -> ()
            n2983 = global write "EV05全局变量1.vi" "流控帧 2"(FALSE ("流控帧 2")) -> ()
            n2984 = local write "消除"(TRUE ("消除")) -> ()
            n2985 = local write "命令"(w4224) -> ()
            n2986 = local write "写?"(FALSE ("写?")) -> ()
          }
          frame #2 {
            n2987 = flat-sequence {
              tunnel: [w4267] -> w4266
              tunnel: w4266 -> [w4274]
              frame #0 {
                n2988 = while {
                  tunnel: [w4268] -> w4267
                  i -> [w4272]
                  stop <- w4269 stop-if-true
                  n2989 = local read "继电器超时处理"() -> (w4268:bool)
                  n2990 = Greater Or Equal?(x=w4272, y=20) -> (x >= y?=w4270:bool)
                  n2991 = Wait Until Next ms Multiple(millisecond multiple=u32 100 ("毫秒倍数")) -> ()  [unwired: 1 out]
                  n2992 = Or(x=w4268, y=w4270) -> (x .or. y?=w4269:bool)
                }
              }
              frame #1 {
                n2993 = case shown="假" w4274 {
                  frame False {
                    n2994 = local read "预充电继电器"() -> (w4275:bool)
                    n2995 = Not(x=w4275) -> (.not. x?=w4276:bool)
                    n2996 = local write "预充电继电器"(w4276) -> ()
                    n2997 = One Button Dialog(message="继电器处理超时" ("消息"), button name ("OK")="是" ("按钮名称（“确定”）")) -> ()  [unwired: 1 out]
                  }
                  frame True {
                  }
                }
              }
            }
          }
        }
      }
      event "加热继电器": Value Change {
        n2998 = event-data() -> ("NewVal"=w4279:bool)  [unwired: 6 out]
        n2999 = stacked-sequence {
          tunnel: w4279 -> [_ w4291 _]
          frame #0 {
            w4282 = FALSE ("继电器超时处理")
            n3000 = local write "继电器超时处理"(w4282) -> ()
            n3001 = local write "正级继电器 5"(w4282) -> ()
            n3002 = local write "主从选择"(enum32{"主板", "从板"}."主板" ("主从选择")) -> ()
          }
          frame #1 {
            n3003 = case shown="假" w4291 {
              selector: w4291 -> [w4305 w4325]
              tunnel: [w4304 w4324] -> w4290
              tunnel: [w4293 w4313] -> w4285
              frame False {
                w4301 = 256.0 ("y")
                w4293 = u32 1 ("命令序号")
                w4304 = u8 192 ("命令")
                n3004 = local read "动作保持时间"() -> (w4302:dbl)
                n3005 = Quotient & Remainder(x=w4302, y=w4301) -> (x-y*floor(x/y)=w4294:dbl, floor(x/y)=w4298:dbl)
                n3006 = Quotient & Remainder(x=w4298, y=w4301) -> (x-y*floor(x/y)=w4295:dbl, floor(x/y)=w4299:dbl)
                n3007 = Quotient & Remainder(x=w4299, y=w4301) -> (x-y*floor(x/y)=w4296:dbl, floor(x/y)=w4300:dbl)
                n3008 = Quotient & Remainder(x=w4300, y=w4301) -> (x-y*floor(x/y)=w4297:dbl)  [unwired: 1 out]
                n3009 = Boolean To (0,1)(Boolean=w4305) -> (0, 1=w4303:i16)
                n3010 = local read "设备索引号"() -> (w4310:u16)
                n3011 = local read "CAN卡类型"() -> (w4311:u32)
                n3012 = local read "CAN端口"() -> (w4309:u16)
                n3013 = Build Array(i16 4 ("元素"), w4303, w4297, w4296, w4295, w4294, 0.0 ("元素")) -> (w4307:dbl[])
                n3014 = call "多帧发送机制(EV05).vi"("can卡类型"=w4311, "设备索引号"=w4310, "CAN端口"=w4309, "命令"=w4304, "板号"=u8 0, "命令序号"=w4293, "输入数据"=w4307) -> ()  [unwired: 1 in, 12 out]
              }
              frame True {
                w4321 = 256.0 ("y")
                w4313 = u32 1 ("命令序号")
                w4324 = u8 192 ("命令")
                n3015 = local read "动作保持时间"() -> (w4322:dbl)
                n3016 = Quotient & Remainder(x=w4322, y=w4321) -> (x-y*floor(x/y)=w4314:dbl, floor(x/y)=w4318:dbl)
                n3017 = Quotient & Remainder(x=w4318, y=w4321) -> (x-y*floor(x/y)=w4315:dbl, floor(x/y)=w4319:dbl)
                n3018 = Quotient & Remainder(x=w4319, y=w4321) -> (x-y*floor(x/y)=w4316:dbl, floor(x/y)=w4320:dbl)
                n3019 = Quotient & Remainder(x=w4320, y=w4321) -> (x-y*floor(x/y)=w4317:dbl)  [unwired: 1 out]
                n3020 = Boolean To (0,1)(Boolean=w4325) -> (0, 1=w4323:i16)
                n3021 = local read "设备索引号"() -> (w4330:u16)
                n3022 = local read "CAN卡类型"() -> (w4331:u32)
                n3023 = local read "CAN端口"() -> (w4329:u16)
                n3024 = Build Array(i16 4 ("元素"), w4323, w4317, w4316, w4315, w4314, 0.0 ("元素")) -> (w4327:dbl[])
                n3025 = call "多帧发送机制(EV05).vi"("can卡类型"=w4331, "设备索引号"=w4330, "CAN端口"=w4329, "命令"=w4324, "板号"=u8 0, "命令序号"=w4313, "输入数据"=w4327) -> ()  [unwired: 1 in, 12 out]
              }
            }
            n3026 = local write "命令序号"(w4285) -> ()
            n3027 = local write "清BUFF"(FALSE ("清BUFF")) -> ()
            n3028 = local write "命令"(w4290) -> ()
            n3029 = local write "控制1"(TRUE ("控制1")) -> ()
            n3030 = global write "EV05全局变量1.vi" "流控帧 2"(FALSE ("流控帧 2")) -> ()
            n3031 = local write "写?"(FALSE ("写?")) -> ()
            n3032 = local write "消除"(TRUE ("消除")) -> ()
          }
          frame #2 {
            n3033 = flat-sequence {
              tunnel: [w4333] -> w4332
              tunnel: w4332 -> [w4340]
              frame #0 {
                n3034 = while {
                  tunnel: [w4334] -> w4333
                  i -> [w4338]
                  stop <- w4335 stop-if-true
                  n3035 = local read "继电器超时处理"() -> (w4334:bool)
                  n3036 = Greater Or Equal?(x=w4338, y=20) -> (x >= y?=w4336:bool)
                  n3037 = Wait Until Next ms Multiple(millisecond multiple=u32 100 ("毫秒倍数")) -> ()  [unwired: 1 out]
                  n3038 = Or(x=w4334, y=w4336) -> (x .or. y?=w4335:bool)
                }
              }
              frame #1 {
                n3039 = case shown="假" w4340 {
                  frame False {
                    n3040 = local read "加热继电器"() -> (w4341:bool)
                    n3041 = Not(x=w4341) -> (.not. x?=w4342:bool)
                    n3042 = local write "加热继电器"(w4342) -> ()
                    n3043 = One Button Dialog(message="继电器处理超时" ("消息"), button name ("OK")="是" ("按钮名称（“确定”）")) -> ()  [unwired: 1 out]
                  }
                  frame True {
                  }
                }
              }
            }
          }
        }
      }
      event "充电继电器": Value Change {
        n3044 = event-data() -> ("NewVal"=w4345:bool)  [unwired: 6 out]
        n3045 = stacked-sequence {
          tunnel: w4345 -> [_ w4357 _]
          frame #0 {
            w4348 = FALSE ("继电器超时处理")
            n3046 = local write "主从选择"(enum32{"主板", "从板"}."主板" ("主从选择")) -> ()
            n3047 = local write "继电器超时处理"(w4348) -> ()
            n3048 = local write "正级继电器 4"(w4348) -> ()
          }
          frame #1 {
            n3049 = case shown="假" w4357 {
              selector: w4357 -> [w4371 w4391]
              tunnel: [w4370 w4390] -> w4356
              tunnel: [w4359 w4379] -> w4351
              frame False {
                w4367 = 256.0 ("y")
                w4359 = u32 1 ("命令序号")
                w4370 = u8 192 ("命令")
                n3050 = local read "动作保持时间"() -> (w4368:dbl)
                n3051 = Quotient & Remainder(x=w4368, y=w4367) -> (x-y*floor(x/y)=w4360:dbl, floor(x/y)=w4364:dbl)
                n3052 = Quotient & Remainder(x=w4364, y=w4367) -> (x-y*floor(x/y)=w4361:dbl, floor(x/y)=w4365:dbl)
                n3053 = Quotient & Remainder(x=w4365, y=w4367) -> (x-y*floor(x/y)=w4362:dbl, floor(x/y)=w4366:dbl)
                n3054 = Quotient & Remainder(x=w4366, y=w4367) -> (x-y*floor(x/y)=w4363:dbl)  [unwired: 1 out]
                n3055 = Boolean To (0,1)(Boolean=w4371) -> (0, 1=w4369:i16)
                n3056 = local read "设备索引号"() -> (w4376:u16)
                n3057 = local read "CAN卡类型"() -> (w4377:u32)
                n3058 = local read "CAN端口"() -> (w4375:u16)
                n3059 = Build Array(i16 5 ("元素"), w4369, w4363, w4362, w4361, w4360, 0.0 ("元素")) -> (w4373:dbl[])
                n3060 = call "多帧发送机制(EV05).vi"("can卡类型"=w4377, "设备索引号"=w4376, "CAN端口"=w4375, "命令"=w4370, "板号"=u8 0, "命令序号"=w4359, "输入数据"=w4373) -> ()  [unwired: 1 in, 12 out]
              }
              frame True {
                w4387 = 256.0 ("y")
                w4379 = u32 1 ("命令序号")
                w4390 = u8 192 ("命令")
                n3061 = local read "动作保持时间"() -> (w4388:dbl)
                n3062 = Quotient & Remainder(x=w4388, y=w4387) -> (x-y*floor(x/y)=w4380:dbl, floor(x/y)=w4384:dbl)
                n3063 = Quotient & Remainder(x=w4384, y=w4387) -> (x-y*floor(x/y)=w4381:dbl, floor(x/y)=w4385:dbl)
                n3064 = Quotient & Remainder(x=w4385, y=w4387) -> (x-y*floor(x/y)=w4382:dbl, floor(x/y)=w4386:dbl)
                n3065 = Quotient & Remainder(x=w4386, y=w4387) -> (x-y*floor(x/y)=w4383:dbl)  [unwired: 1 out]
                n3066 = Boolean To (0,1)(Boolean=w4391) -> (0, 1=w4389:i16)
                n3067 = local read "设备索引号"() -> (w4396:u16)
                n3068 = local read "CAN卡类型"() -> (w4397:u32)
                n3069 = local read "CAN端口"() -> (w4395:u16)
